vi "DWE Property nodes testing.vi"() -> ()   [LabVIEW 2014]
panel:
  in  "Tab Control 3":enum32{"Page 1", "Page 2"}(tab)
  in  "Page 1 Color":u32(colorbox)=16750592
  in  "stop":bool
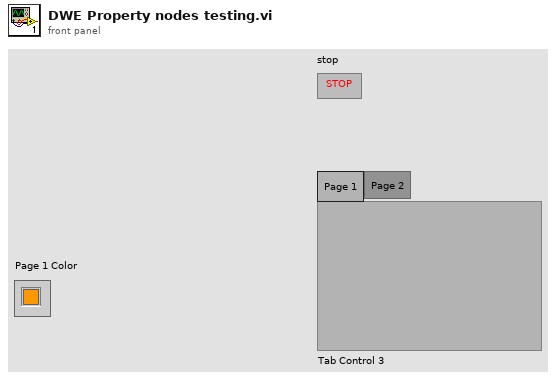
[diagram p1: front panel]
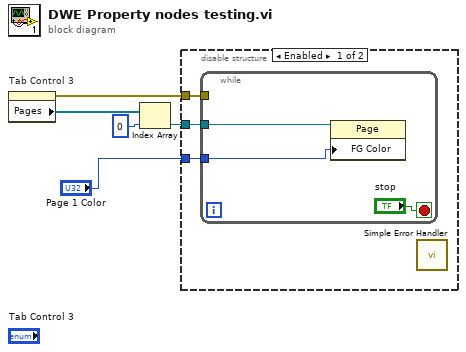
[diagram p0: block diagram]
diagram:
  n1 = property on="Tab Control 3" class="TabCtl (strict)"() -> (error out=w3:errorcluster, "Pages"=w2:refnum<vi>[])  [unwired: 2 in, 1 out]
  n2 = Index Array(array=w2, index=0) -> (element=w4:refnum<vi>)
  n3 = disable-structure shown="Enabled" {
    disable-tunnel: w4 -> [w8 _]
    disable-tunnel: w3 -> [w7 _]
    disable-tunnel: "Page 1 Color" -> [w6 _]
    frame Enabled {
      n4 = while {
        tunnel: w7 -> [_]
        tunnel: w8 -> [w10]
        tunnel: w6 -> [w9]
        stop <- "stop" stop-if-true
        n5 = property class="Page"(reference=w10, "FG Color"=w9) -> ()  [unwired: 1 in, 2 out]
      }
      n6 = call <vilib>:"Simple Error Handler.vi"() -> ()  [unwired: 5 in, 5 out]
    }
    frame Disabled {
    }
  }
